vi "Gradient Read Single.vi"(8 "error in":errorcluster, 9 "Channel Index":i32=1, 11 "Power Gradient in":refnum<class "Power Gradient.lvclass">) -> (0 "error out":errorcluster, 1 "Changed or First Call?":bool, 2 "Power SP":dbl, 3 "Power Gradient out":refnum<class "Power Gradient.lvclass">)   [LabVIEW 2023, in "Power Gradient.lvclass"]
uses:
  Power Gradient.lvclass
  Parents/Gradient/Gradient.lvclass
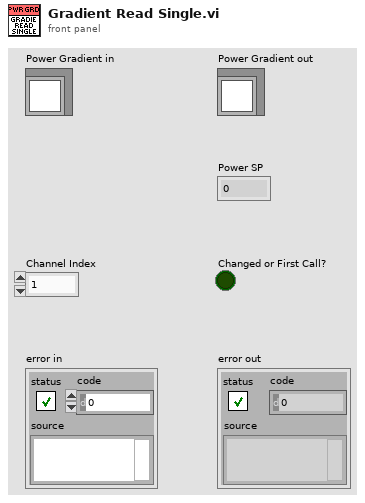
[diagram p1: front panel]
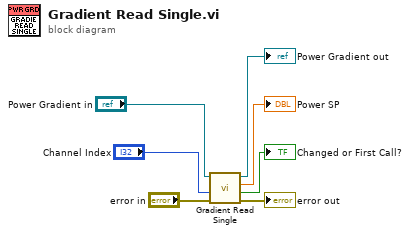
[diagram p0: block diagram]
diagram:
  n1 = call-parent "Gradient Read Single.vi"("error in"="error in", "Channel Index"="Channel Index", "Gradient in"="Power Gradient in") -> ("error out"=→"error out":errorcluster, "Changed or First Call?"=→"Changed or First Call?":bool, "Current SP"=→"Power SP":dbl, "Gradient out"=→"Power Gradient out":refnum<class "Power Gradient.lvclass">)  [unwired: 5 in]
